vi "5.10 Blue Filter Lower Limit Control System.vi"(8 "Reasonable Guess":dbl=40.0, 9 "Override":bool=TRUE, 10 "Blue":cluster{"Lower value":i32, "Upper value":i32}={"Lower value"=0, "Upper value"=255} {"Upper value" scale=0.0..255.0; "Lower value" scale=0.0..255.0}, 11 "Incoming Control Signals":dbl[][](array[numeric])) -> (2 "Blue Out":cluster{"Lower value":i32, "Upper value":i32}={"Lower value"=0, "Upper value"=255} {"Upper value" scale=0.0..255.0; "Lower value" scale=0.0..255.0})   [LabVIEW 2010]
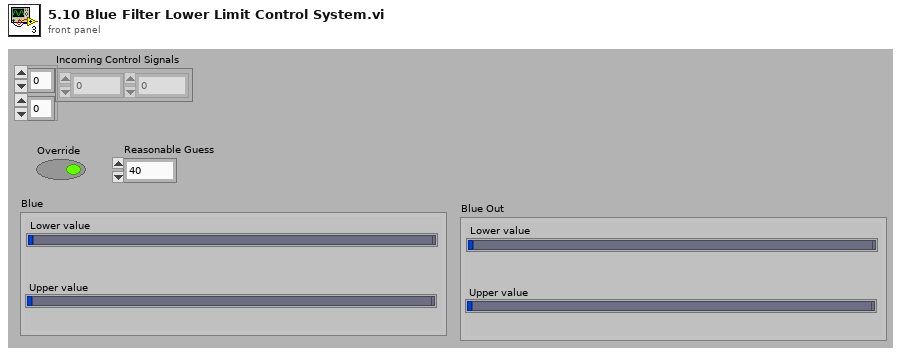
[diagram p1: front panel]
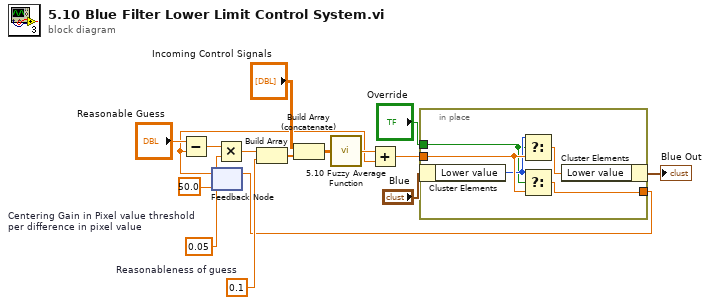
[diagram p0: block diagram]
diagram:
  w10 = 0.1  # Reasonableness of guess
  w12 = 0.05  # Centering Gain in Pixel value threshold per difference in pixel value
  n1 = feedback #1(50.0) -> (w4:dbl)
  n2 = Subtract(x="Reasonable Guess", y=w4) -> (x-y=w13:dbl)
  n3 = Multiply(x=w13, y=w12) -> (x*y=w11:dbl)
  n4 = Build Array(w11, w10) -> (w9:dbl[])
  n5 = Build Array (concatenate)("Incoming Control Signals", w9) -> (w16:dbl[][])
  n6 = call "5.10 Fuzzy Average Function.vi"("Input Control Certainty Array"=w16) -> ("Output Control Value"=w15:dbl)
  n7 = Add(x=w15, y=w4) -> (x+y=w2:dbl)
  n8 = in-place {
    in-place-border: w2 -> [w20]
    in-place-border: "Override" -> [w18]
    in-place-border: [w17] -> w1
    n9 = in-place-cluster #2("Blue") -> ("Lower value"=w19:i32)
    n10 = Select(t=w19, s=w18, f=w20) -> (s? t:f=w21:dbl)
    n11 = Select(t=w19, s=w18, f=w20) -> (s? t:f=w17:dbl)
    n12 = in-place-cluster #2("Lower value"=w21) -> (→"Blue Out":cluster{"Lower value":i32, "Upper value":i32})
  }
  n13 = feedback-in #1(w1) -> ()
